vi "LVClass_ModalCoef equalize AB.vi"(0 "ModalCoef Dest in":refnum<class "ModalCoef.lvclass">, 5 "ModalCoef Source in":refnum<class "ModalCoef.lvclass">, 11 "error in (no error)":errorcluster) -> (4 "ModalCoef Dest out":refnum<class "ModalCoef.lvclass">, 6 "ModalCoef Source out":refnum<class "ModalCoef.lvclass">, 15 "error out":errorcluster)   [LabVIEW 2020, in "ModalCoef.lvclass"]
doc: "ModalCoef constructor.\n\n--------------------------------------------------------------------------------\n\n<B>ModalCoefIn </B> : Constant Pointer to ModalCoef object.\n<B>ModalCoefOut </B> : Constant Pointer to ModalCoef object.\n<B>TypePhase </B> : TypePhase Phase mode reconstruction.\n<B>ErrorIn </B> : Error\n<B>ErrorOut </B> : Error\n\n--------------------------------------------------------------------------------"
uses:
  ModalCoef.lvclass
  Handle creation.ctl
  ModalCoef.lvclass/ModalCoef.ctl
  LVClass_ModalCoef Read ModalCoef.vi
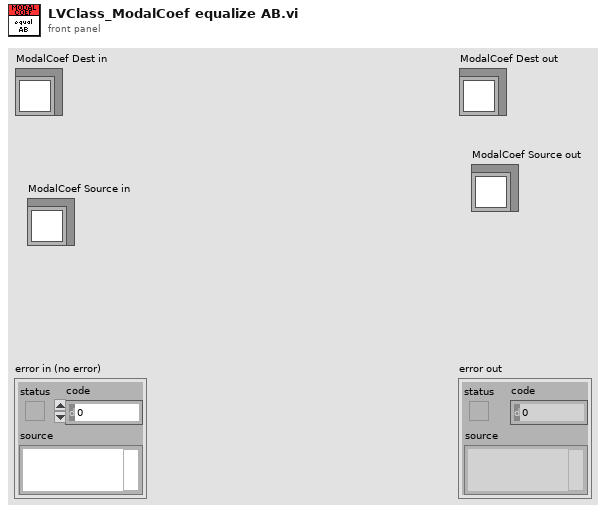
[diagram p1: front panel]
types:
  T1 = typedef "Handle creation.ctl" = enum16{"By ctor", "By write function"}
  T2 = typedef "ClassID.ctl" = i64
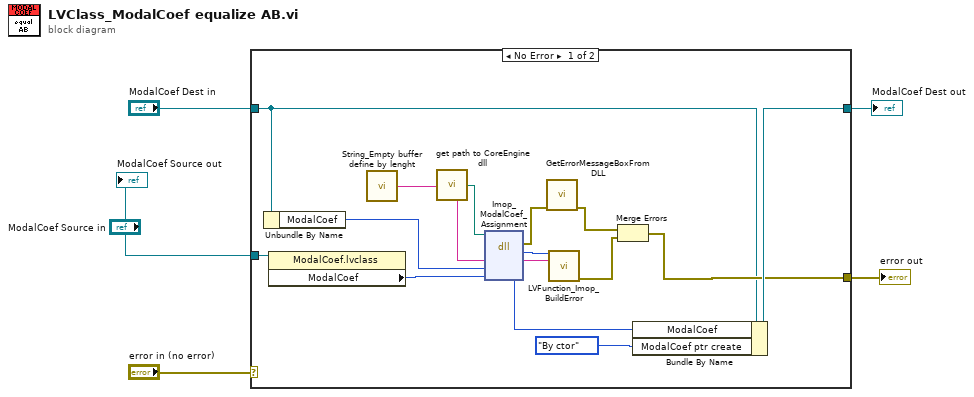
[diagram p0: block diagram]
diagram:
  n1 = case shown="No Error" "error in (no error)" {
    selector: "error in (no error)" -> [_ w22]
    tunnel: [w10 w22] -> w4
    tunnel: [w13 w21] -> w2
    tunnel: "ModalCoef Dest in" -> [w7 w21]
    tunnel: "ModalCoef Source in" -> [w9 _]
    frame No Error {
      n2 = Unbundle By Name(w7) -> ("ModalCoef"=w6:T2)
      n3 = property class="ModalCoef.lvclass"(reference=w9) -> ("ModalCoef"=w8:T2)  [unwired: 1 in, 2 out]
      n4 = call "String_Empty buffer define by lenght.vi"() -> ("Empty buffer"=w20:string)  [unwired: 1 in]
      n5 = call "get path to CoreEngine dll.vi"() -> ("path to wavekit library"=w17:path)  [unwired: 14 in, 1 out]
      n6 = dll-call lib="D:/soft/HASO_v3/SVN_trunk/ImOpCoreEngine4_LV2011/DLLs/c_interface_vc100.dll" fn="Imop_ModalCoef_Assignment"(path in=w17, "message"=w20, "ModalCoef Dest"=w6, "ModalCoef Source"=w8) -> (error out=w16:errorcluster, "return type"=w18:i32, "message"=w19:string, "ModalCoef Dest"=w15:i64)  [unwired: 3 in, 1 out]
      n7 = call "GetErrorMessageBoxFromDLL.vi"("error IN"=w16) -> ("error OUT"=w12:errorcluster)  [unwired: 10 in]
      n8 = call "LVFunction_Imop_BuildError.vi"("code"=w18, "String to Prepend to source (\"\")"=w19) -> ("error out"=w11:errorcluster)  [unwired: 13 in]
      n9 = Merge Errors(w12, w11) -> (w10:errorcluster)
      n10 = Bundle By Name(cluster=w7, "ModalCoef"=w15, "ModalCoef ptr create"=Handle_creation."By ctor" ("Pupil ptr create")) -> (w13:refnum<class "ModalCoef.lvclass">)
    }
    frame Error {
    }
  }
  "error out" <- w4
  "ModalCoef Dest out" <- w2
  "ModalCoef Source out" <- "ModalCoef Source in"
